vi "Msg.Event.Register.vi"(8 "Error (in)":errorcluster, 11 "Msg.Event.Ref":T1) -> (0 "Error (out)":errorcluster, 2 "Event Registration Refnum":T2, 3 "Msg.Event.Ref (out)":T1)   [LabVIEW 2023, in "MessagingModule.lvlib"]
doc: "Used to create a register a user event."
uses:
  Msg.Event.Ref.ctl
  Msg.Data.ctl
  Msg.Event.RegRef.ctl
  MessagingModule.lvlib
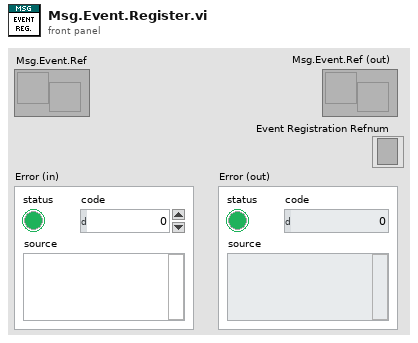
[diagram p1: front panel]
types:
  T1 = typedef "MessagingModule.lvlib/Msg.Event.Ref.ctl" = refnum<user-event>
  T2 = typedef "MessagingModule.lvlib/Msg.Event.RegRef.ctl" = refnum<event-registration>
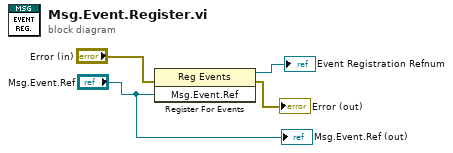
[diagram p0: block diagram]
diagram:
  n1 = register-events(error in="Error (in)", "Msg.Event.Ref") -> (reference out=→"Event Registration Refnum":refnum<event-registration>, error out=→"Error (out)":errorcluster)  [unwired: 1 in]
  "Msg.Event.Ref (out)" <- "Msg.Event.Ref"
